vi "Set Bitmap.vi"(8 "error in (no error)":errorcluster, 10 "Bitmap":u32[][](array[numeric]), 11 "Glyph Canvas in":refnum<class "Tree Control Canvas.lvclass">) -> (0 "error out":errorcluster, 3 "Glyph Canvas out":refnum<class "Tree Control Canvas.lvclass">)   [LabVIEW 2020, in "Glyph Drawer.lvlib" / "Tree Control Canvas.lvclass"]
uses:
  Tree Control Canvas.lvclass
  Tree Control Canvas.lvclass/Tree Control Canvas.ctl
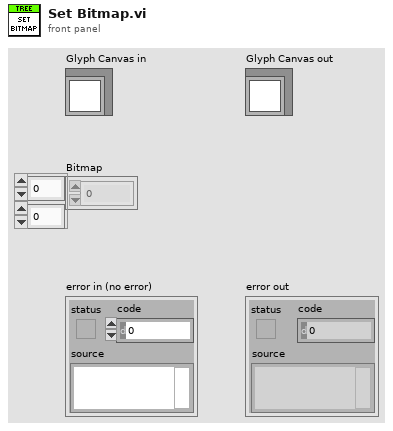
[diagram p1: front panel]
types:
  T1 = typedef "imagedata.ctl" = cluster{"image type":i32, "image depth":i32, "image":u8[], "mask":u8[], "colors":u32[], "Rectangle":cluster{"left":i16, "top":i16, "right":i16, "bottom":i16}}
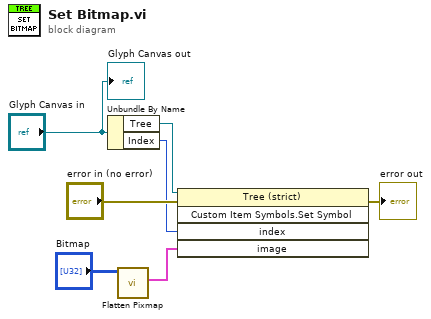
[diagram p0: block diagram]
diagram:
  n1 = Unbundle By Name("Glyph Canvas in") -> ("Tree"=w6:refnum<vi>, "Index"=w2:i32)
  n2 = call <vilib>:"Flatten Pixmap.vi"("24-bit pixmap"="Bitmap") -> ("image data"=w1:T1)  [unwired: 10 in]
  n3 = invoke class="Tree (strict)" method="Custom Item Symbols.Set Symbol"(reference=w6, error in="error in (no error)", "index"=w2, "image"=w1) -> (error out=→"error out":errorcluster)  [unwired: 1 in, 4 out]
  "Glyph Canvas out" <- "Glyph Canvas in"
